vi "Create DataLog List.vi"(8 "error in (no error)":errorcluster, 10 "Log List":refnum<vi>, 11 "Refnum in":T1) -> (0 "error out":errorcluster)   [LabVIEW 2018]
doc: "creates ProjectConfig table in existing database."
uses:
  <vilib>/addons/database/Connection.llb/Conn ObjectReference.ctl
  <vilib>/addons/database/Auxilliary.llb/DB Tools Column Info.ctl
  <vilib>/addons/database/Auxilliary.llb/DB Tools DataTypes.ctl
  <vilib>/addons/database/NI_Database_API.lvlib
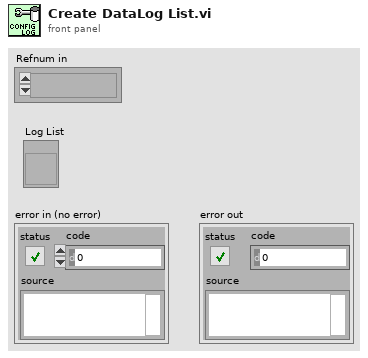
[diagram p1: front panel]
types:
  T1 = typedef "NI_Database_API.lvlib/Conn ObjectReference.ctl" = refnum<k1>
  T2 = typedef "NI_Database_API.lvlib/DB Tools Column Info.ctl" = cluster{"column name":string, "data type":T3, "size":i32, "allow null?":bool}
  T3 = typedef "NI_Database_API.lvlib/DB Tools DataTypes.ctl" = enum16{"String", "Long (I32)", "Single (SGL)", "Double (DBL)", "Date/Time", "Binary"}
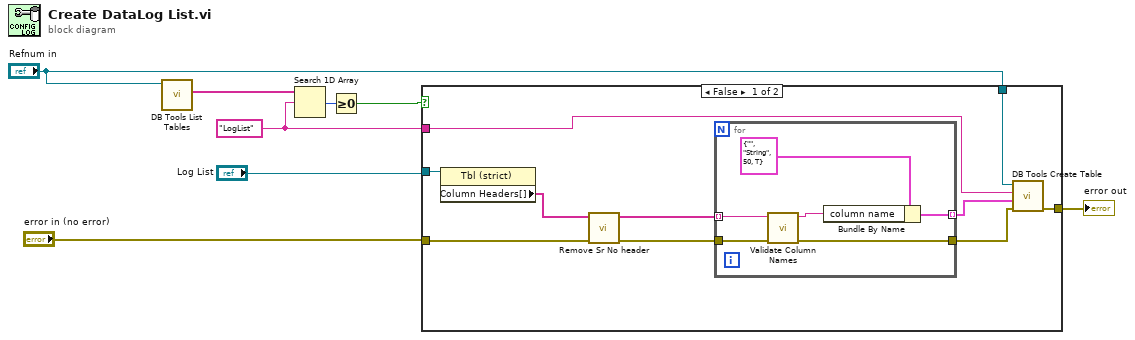
[diagram p0: block diagram]
diagram:
  w4 = "LogList" ("table")
  n1 = call <vilib>:"DB Tools List Tables.vi"("connection reference"="Refnum in") -> ("tables"=w5:string[])  [unwired: 4 in, 2 out]
  n2 = Search 1D Array(1D array=w5, element=w4) -> (index of element=w3:i32)  [unwired: 1 in]
  n3 = Greater Or Equal To 0?(x=w3) -> (x >= 0?=w2:bool)
  n4 = case shown="False" w2 {
    tunnel: "Log List" -> [w11 _]
    tunnel: "error in (no error)" -> [w16 w24]
    tunnel: [w15 w24] -> w7
    tunnel: "Refnum in" -> [w13 _]
    tunnel: w4 -> [w12 _]
    frame False {
      n5 = property class="Tbl (strict)"(reference=w11) -> ("Column Headers[]"=w10:string[])  [unwired: 1 in, 2 out]
      n6 = call "Remove Sr No header.vi"("Column Headers[] in"=w10) -> ("Column Headers[] out"=w9:string[])  [unwired: 10 in]
      n7 = for {
        tunnel: [w23] -> w14 mode=indexing
        tunnel: w16 -> [w21]
        tunnel: [w20] -> w17
        tunnel: w9 -> [w18] mode=indexing
        n8 = call "Validate Column Names.vi"("error in (no error)"=w21, "Label.Text"=w18) -> ("error out"=w20:errorcluster, "result string"=w22:string)  [unwired: 8 in]
        n9 = Bundle By Name(cluster=T2 {"column name"="", "data type"=enum."String", "size"=50, "allow null?"=TRUE} ("column information"), "column name"=w22) -> (w23:T2)
      }
      n10 = call <vilib>:"DB Tools Create Table.vi"("error in (no error)"=w17, "column information"=w14, "table"=w12, "connection reference"=w13) -> ("error out"=w15:errorcluster)  [unwired: 4 in, 1 out]
    }
    frame True {
    }
  }
  "error out" <- w7
